vi "Solve2.vi"(8 "Error In":errorcluster, 11 "object in":refnum<class "2024_18.lvclass">) -> (0 "Error Out":errorcluster, 2 "Result":u64, 3 "object out":refnum<class "2024_18.lvclass">)   [LabVIEW 2023, in "2024_18.lvclass"]
uses:
  2024_18.lvclass
  Common/AOC_XY(I32).ctl
  2024_18.lvclass/2024_18.ctl
panel:
  out "element":T1
  out "size(s)":i32
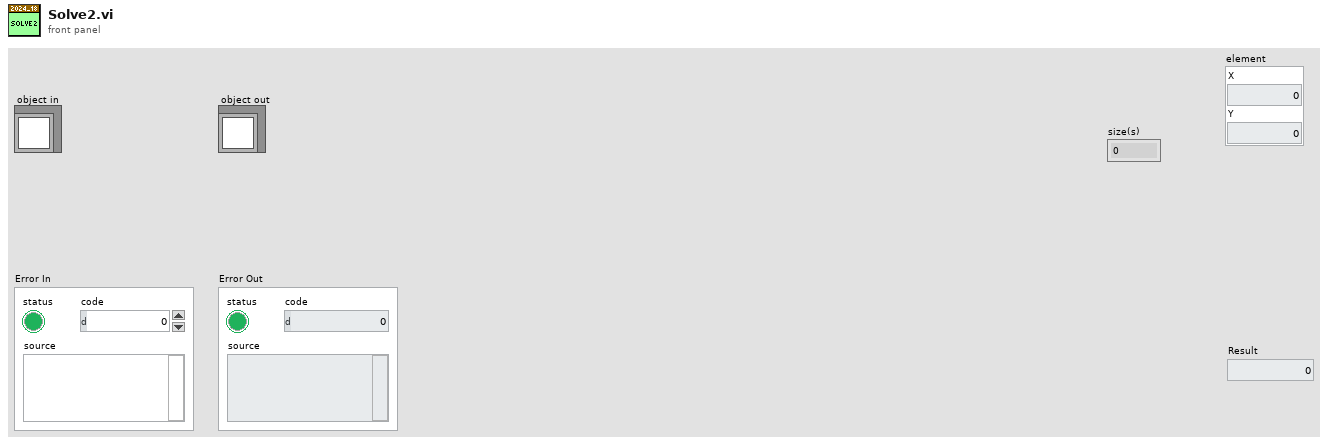
[diagram p1: front panel]
types:
  T1 = typedef "AOC_XY(I32).ctl" = cluster{"X":i32, "Y":i32}
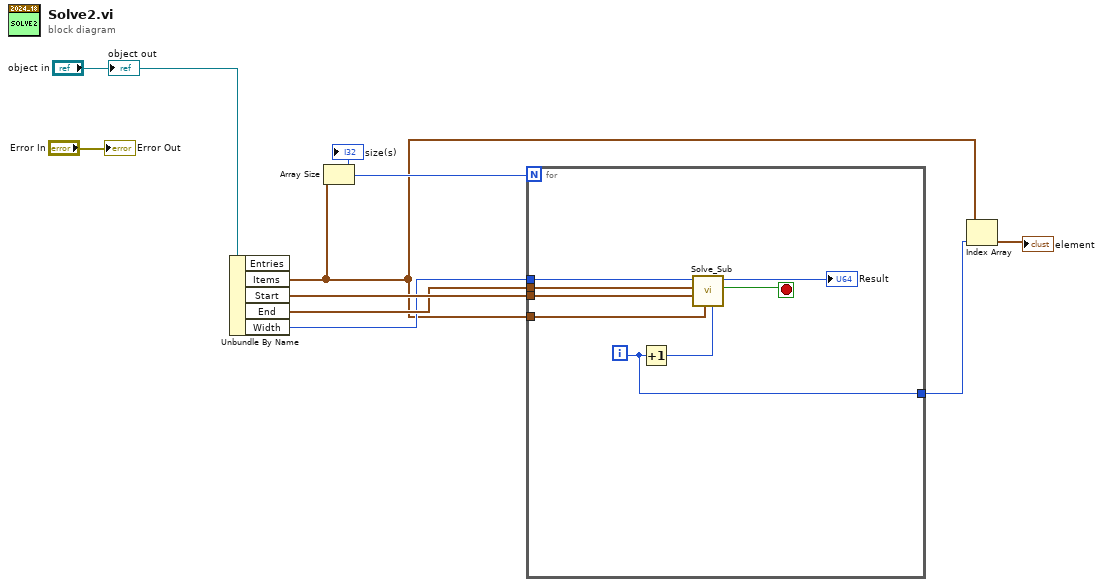
[diagram p0: block diagram]
diagram:
  n1 = Unbundle By Name("object in") -> ("Items"=w3:T1[], "Start"=w8:T1, "End"=w7:T1, "Width"=w6:i32)  [unwired: 1 out]
  n2 = Array Size(array=w3) -> (size(s)=w4:i32)
  "size(s)" <- w4
  n3 = for {
    N: w4 -> [_]
    tunnel: w8 -> [w17]
    tunnel: w7 -> [w16]
    tunnel: w6 -> [w15]
    tunnel: w3 -> [w14]
    tunnel: [w10] -> w1
    i -> [w10]
    stop <- w12 stop-if-true
    n4 = Increment(x=w10) -> (x+1=w13:i32)
    n5 = call "Solve_Sub.vi"("Entries"=w13, "Items"=w14, "Start"=w17, "End"=w16, "Width/Height"=w15) -> ("key not found?"=w12:bool, "Cost"=→"Result":u64)  [unwired: 4 in, 1 out]
  }
  n6 = Index Array(array=w3, index=w1) -> (element=→"element":T1)
  "Error Out" <- "Error In"
  "object out" <- "object in"
